vi "Basic.vi"() -> (0 "error out":errorcluster)   [LabVIEW 2019, in "GettingStarted_5785_Host.lvlib"]
uses:
  GettingStarted_5785_Host.lvlib
  <vilib>/userDefined/Silver/nirio_resource_slv.ctl
  <instrlib>/FlexRIO/API/Host/v1/NI FlexRIO/API/Reference Clock Source.ctl
  Upconversion Mode.ctl
  <instrlib>/FlexRIO/API/Host/v1/NI FlexRIO/API/Configure Reference Clock.vi
  <instrlib>/FlexRIO/API/Host/v1/NI FlexRIO/API/Get Property Reference - Fpga Small.vi
  <instrlib>/FlexRIO/API/Host/v1/NI FlexRIO/API/Configure Analog Start Trigger.vi
  <instrlib>/FlexRIO/API/Host/v1/NI FlexRIO/API/Configure Digital Edge Start Trigger.vi
  <instrlib>/FlexRIO/API/Host/v1/NI FlexRIO/API/Configure Immediate Start Trigger.vi
  <instrlib>/FlexRIO/API/Host/v1/NI FlexRIO/API/Read Stream 1D WDT.vi
  <vilib>/measure/matone.llb/Extract Single Tone Information N Chan (CDB).vi
  <vilib>/measure/maspectr.llb/FFT Power Spectrum and PSD for N Chan (CDB).vi
  <vilib>/FPGAPlugInAG/Dynamic/niLvFpga_Close_Dynamic.vi
  <vilib>/rvi/interface/nirviCloseFPGA/nirviCloseFPGA.xnode
  <instrlib>/FlexRIO/API/Host/v1/NI FlexRIO API v1.lvlib
  <resource>/objmgr/niflexrioapiStream.rc
  <vilib>/measure/NI_MAPro.lvlib
panel:
  in  "DUC Freq Shift (Hz)":dbl format="%#_4p"
  in  "DDC Freq Shift (Hz)":dbl format="%#_4p"
  in  "IQ Enabled":bool
  in  "DDC Enabled":bool
  in  "processing mode":T1=enum."None, Two Channels"
  out "AO num Samples":i32=160
  in  "waveform config":T2(array[cluster])=[{"Frequency (Hz)"=500000000.0, "Amplitude (V)"=0.2, "Phase (Deg)"=0.0}, {"Frequency (Hz)"=500000000.0, "Amplitude (V)"=0.20000000000000004, "Phase (Deg)"=0.0}] {"Phase (Deg)" format="%.2p"; "Amplitude (V)" format="%0.2p"; "Frequency (Hz)" format="%0.2p"}
  in  "reference clock source":T3 items=["Default", "Onboard", "PXI_Clk10", "External", "None", "Baseboard Reference"]
  in  "Update Waveform":bool caption="Download AO Waveforms"
  out "Sample Rate":dbl=3200000000.0 format="%#_6p"
  in  "ADC Interleaving Factor":i32=1 min=0 max=2 step=1
  in  "AI num samples":u64=320 step=32
  in  "AI channels":string="AI0,AI1"
  out "Device Power":dbl(slide)=32.59 scale=-1.0..58.0 scale format="%#_3p"
  out "FPGA Temperature":dbl(slide)=48.0 scale=0.0..100.0 scale format="%#_3p"
  in  "Trigger Type":enum32{"Immediate", "Analog", "Digital"}(tab)
  in  "trigger channel":string="AI0"
  in  "rising edge?":bool=TRUE
  in  "level (V)":dbl format="%#_3p"
  in  "hysteresis (V)":dbl=0.01 format="%#_3p"
  in  "digital trigger source":string(combo)
  in  "stop":bool
  in  "Bitfile path":path=path "C:/Repos/bsherman-sandbox/CogRF/5785 Measurements/Common/Original 5785 Example/FPGA Bitfiles/PXIe_5785_KU060.lvbitx"
  in  "Waveform Tab Control":T4(tab)
  out "Waveform Graph":waveform(dbl)[](graph)=[{"t0"=timestamp(0 s since 1904-01-01), "dt"=3.125e-10, "Y"=array[320 elements]}, {"t0"=timestamp(0 s since 1904-01-01), "dt"=3.125e-10, "Y"=array[320 elements]}]
  out "FFT":cluster{"f0":dbl, "df":dbl, "magnitude":dbl[]}[](graph) caption="Waveform Graph"
  out "detected frequencies":dbl[](array[numeric])=[555552707.7834543, 1412702117.9341562] format="%_4p"
  out "AO Out":waveform(dbl)[](graph)=[{"t0"=timestamp(0 s since 1904-01-01), "dt"=3.125e-10, "Y"=[0.0, 0.16629392246050906, 0.1847759065022574, 0.03901806440322561, -0.1414213562373095, -0.19615705608064604, -0.07653668647301802, 0.11111404660392049, 0.2, 0.11111404660392035, -0.07653668647301787, -0.19615705608064607, -0.14142135623730956, 0.03901806440322578, 0.18477590650225734, 0.16629392246050892, 0.0, -0.16629392246050909, -0.18477590650225734, -0.03901806440322547, 0.14142135623730956, 0.196157056080646, 0.07653668647301785, -0.11111404660392055, -0.19999999999999996, -0.11111404660392023, 0.07653668647301798, 0.19615705608064604, 0.1414213562373094, -0.03901806440322589, -0.18477590650225728, -0.1662939224605088, 5.551115123125783e-17, 0.16629392246050909, 0.18477590650225723, 0.03901806440322533, -0.14142135623730945, -0.19615705608064585, -0.07653668647301788, 0.11111404660392057, 0.1999999999999999, 0.11111404660392012, -0.07653668647301798, -0.196157056080646, -0.14142135623730936, 0.03901806440322589, 0.18477590650225725, 0.16629392246050878, -2.7755575615628914e-17, -0.16629392246050906, -0.18477590650225725, -0.03901806440322536, 0.14142135623730942, 0.19615705608064593, 0.07653668647301794, -0.11111404660392066, -0.1999999999999999, -0.11111404660392014, 0.07653668647301792, 0.19615705608064604, 0.14142135623730945, -0.039018064403225916, -0.18477590650225728, -0.1662939224605088, 0.0, 0.16629392246050914, 0.18477590650225728, 0.03901806440322533, -0.14142135623730945, -0.19615705608064596, -0.07653668647301792, 0.11111404660392063, 0.1999999999999999, 0.11111404660392017, -0.07653668647301792, -0.1961570560806461, -0.14142135623730945, 0.039018064403226, 0.18477590650225728, 0.1662939224605088, 0.0, -0.1662939224605092, -0.18477590650225728, -0.039018064403225305, 0.14142135623730945, 0.196157056080646, 0.07653668647301792, -0.11111404660392071, -0.1999999999999999, -0.11111404660392012, 0.07653668647301792, 0.19615705608064615, 0.14142135623730945, -0.039018064403226055, -0.18477590650225728, -0.1662939224605088, 0.0, 0.16629392246050925, 0.18477590650225728, 0.039018064403225305, -0.14142135623730945, -0.19615705608064601, -0.07653668647301792, 0.11111404660392074, 0.1999999999999999, 0.11111404660392014, -0.07653668647301792, -0.1961570560806461, -0.14142135623730945, 0.03901806440322597, 0.18477590650225728, 0.1662939224605088, 0.0, -0.16629392246050914, -0.18477590650225728, -0.03901806440322539, 0.14142135623730945, 0.196157056080646, 0.07653668647301792, -0.1111140466039206, -0.1999999999999999, -0.11111404660392023, 0.07653668647301792, 0.19615705608064604, 0.14142135623730945, -0.03901806440322583, -0.18477590650225728, -0.16629392246050886, 0.0, 0.16629392246050909, 0.18477590650225728, 0.03901806440322539, -0.14142135623730945, -0.19615705608064593, -0.07653668647301792, 0.1111140466039206, 0.1999999999999999, 0.11111404660392019, -0.07653668647301792, -0.19615705608064607, -0.14142135623730945, 0.039018064403225944, 0.18477590650225728, 0.1662939224605088, 0.0, -0.16629392246050914, -0.18477590650225728, -0.03901806440322533, 0.14142135623730945, 0.19615705608064596, 0.07653668647301792, -0.11111404660392063, -0.1999999999999999, -0.11111404660392017, 0.07653668647301792, 0.1961570560806461, 0.14142135623730945, -0.039018064403226, -0.18477590650225728, -0.1662939224605088]}, {"t0"=timestamp(0 s since 1904-01-01), "dt"=3.125e-10, "Y"=[0.0, 0.16629392246050909, 0.1847759065022574, 0.03901806440322561, -0.1414213562373095, -0.19615705608064612, -0.07653668647301798, 0.11111404660392046, 0.20000000000000004, 0.11111404660392046, -0.076536686473018, -0.19615705608064612, -0.1414213562373095, 0.03901806440322561, 0.1847759065022574, 0.1662939224605091, 0.0, -0.166293922460509, -0.1847759065022574, -0.03901806440322575, 0.1414213562373095, 0.1961570560806461, 0.07653668647301802, -0.11111404660392044, -0.2, -0.11111404660392044, 0.07653668647301787, 0.1961570560806461, 0.14142135623730956, -0.03901806440322575, -0.18477590650225734, -0.16629392246050897, 0.0, 0.16629392246050903, 0.18477590650225734, 0.03901806440322558, -0.14142135623730956, -0.196157056080646, -0.07653668647301785, 0.11111404660392044, 0.19999999999999996, 0.11111404660392034, -0.07653668647301798, -0.196157056080646, -0.1414213562373094, 0.039018064403225666, 0.18477590650225728, 0.16629392246050895, -5.551115123125783e-17, -0.166293922460509, -0.18477590650225723, -0.039018064403225555, 0.14142135623730945, 0.19615705608064596, 0.07653668647301788, -0.11111404660392041, -0.1999999999999999, -0.11111404660392037, 0.07653668647301798, 0.196157056080646, 0.14142135623730936, -0.03901806440322561, -0.18477590650225725, -0.16629392246050897, 2.7755575615628914e-17, 0.16629392246050897, 0.18477590650225725, 0.03901806440322564, -0.14142135623730942, -0.19615705608064601, -0.07653668647301794, 0.11111404660392041, 0.1999999999999999, 0.11111404660392041, -0.07653668647301792, -0.19615705608064601, -0.14142135623730945, 0.03901806440322564, 0.18477590650225728, 0.16629392246050897, 0.0, -0.16629392246050897, -0.18477590650225728, -0.03901806440322564, 0.14142135623730945, 0.19615705608064601, 0.07653668647301792, -0.11111404660392041, -0.1999999999999999, -0.11111404660392041, 0.07653668647301792, 0.19615705608064601, 0.14142135623730945, -0.03901806440322564, -0.18477590650225728, -0.16629392246050897, 0.0, 0.16629392246050897, 0.18477590650225728, 0.03901806440322564, -0.14142135623730945, -0.19615705608064601, -0.07653668647301792, 0.11111404660392041, 0.1999999999999999, 0.11111404660392041, -0.07653668647301792, -0.19615705608064601, -0.14142135623730945, 0.03901806440322564, 0.18477590650225728, 0.16629392246050897, 0.0, -0.16629392246050897, -0.18477590650225728, -0.03901806440322564, 0.14142135623730945, 0.19615705608064601, 0.07653668647301792, -0.11111404660392041, -0.1999999999999999, -0.11111404660392041, 0.07653668647301792, 0.19615705608064601, 0.14142135623730945, -0.03901806440322564, -0.18477590650225728, -0.16629392246050897, 0.0, 0.16629392246050897, 0.18477590650225728, 0.03901806440322564, -0.14142135623730945, -0.19615705608064601, -0.07653668647301792, 0.11111404660392041, 0.1999999999999999, 0.11111404660392041, -0.07653668647301792, -0.19615705608064601, -0.14142135623730945, 0.03901806440322564, 0.18477590650225728, 0.16629392246050897, 0.0, -0.16629392246050897, -0.18477590650225728, -0.03901806440322564, 0.14142135623730945, 0.19615705608064601, 0.07653668647301792, -0.11111404660392041, -0.1999999999999999, -0.11111404660392041, 0.07653668647301792, 0.19615705608064601, 0.14142135623730945, -0.03901806440322564, -0.18477590650225728, -0.16629392246050897]}] caption="Waveform Graph"
  out "Limit (W)":dbl=58.0
  out "Power (W)":dbl=32.59
  out "Limit (C)":dbl=96.0
  out "Temp (C)":dbl=48.0 format="%#_4p"
  in  "RIO Device":T5="5785_00"
  # "Overview: Configure an acquisition for a FlexRIO target and transfer the data to the host using the FlexRIO Host API.  Loop an output waveform\nRequirements: FlexRIO\nInstructions: \n 1. Loop AI channels back to AO channels using SMA cables\n 2. Select the RIO Device that corresponds to the FlexRIO target. \n 3. Select the bitfile path that corresponds to your device\n 4. Optionally configure the clocking, stream, and trigger. \n 5. Run the VI"
  # "Resource Configuration"
  # "Clocking configuration"
  # "Input Waveform Configuration"
  # "Device Monitoring"
  # "Output Waveform Configuration"
  # "Digital Upconverter Configuration"
  # "Frequency (Hz)"
  # "Amplitude (V)"
  # "Phase (Deg)"
  # "AO 0"
  # "AO 1"
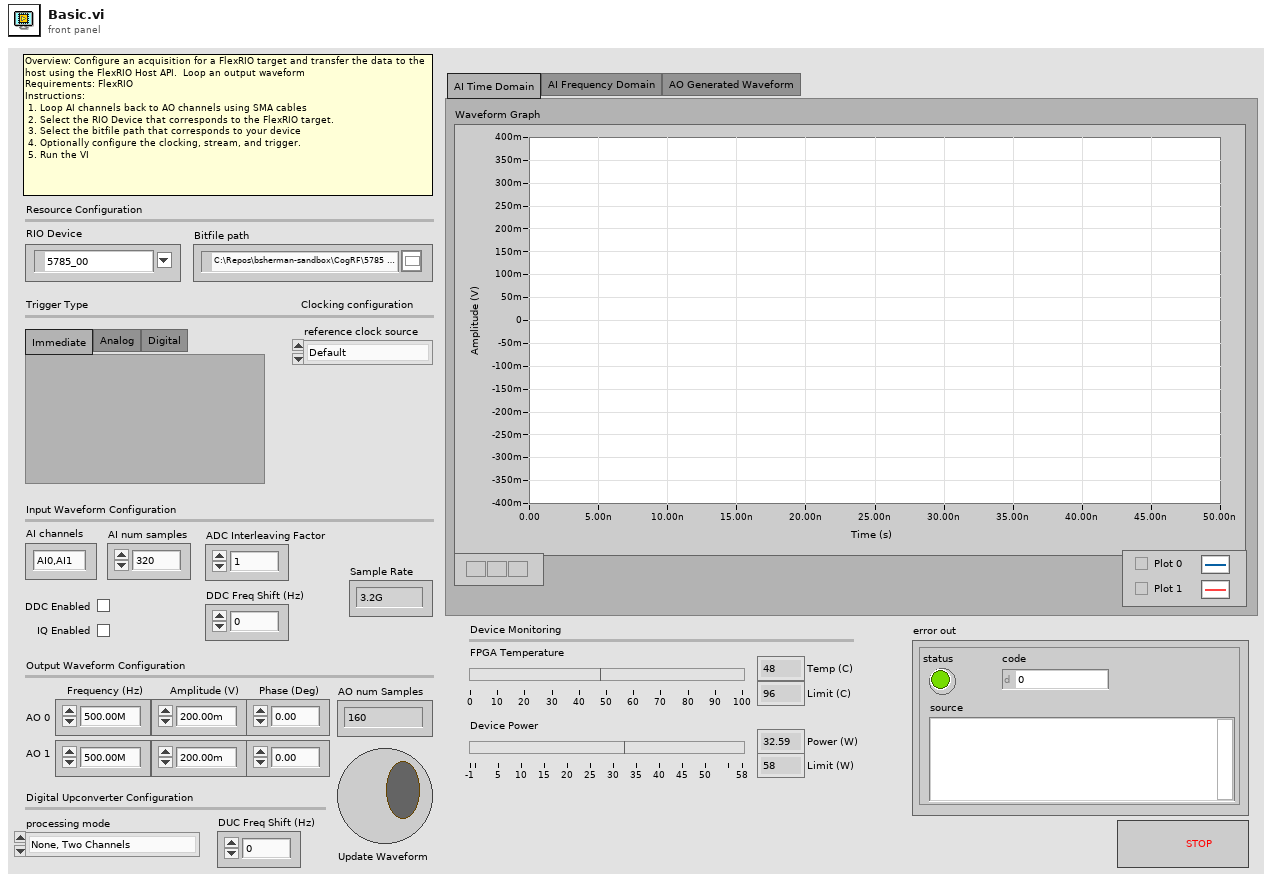
[diagram p1: front panel]
types:
  T1 = typedef "GettingStarted_5785_Host.lvlib/Upconversion Mode.ctl" = enum16{"None, One Channel", "None, Two Channels", "FPGA-only, One Channel", "DAC and FPGA, One Channel", "DAC-only, One Channel"}
  T2 = cluster{"Frequency (Hz)":dbl, "Amplitude (V)":dbl, "Phase (Deg)":dbl}[]
  T3 = typedef "NI FlexRIO API v1.lvlib/Reference Clock Source.ctl" = i32
  T4 = enum32{"AI Time Domain", "AI Frequency Domain", "AO Generated Waveform"}
  T5 = typedef "nirio_resource_slv.ctl" = tag
  T6 = cluster{"averaging mode":enum16{"No averaging", "Vector averaging", "RMS averaging", "Peak hold"}, "weighting mode":enum16{"Linear", "Exponential"}, "number of averages":u32}
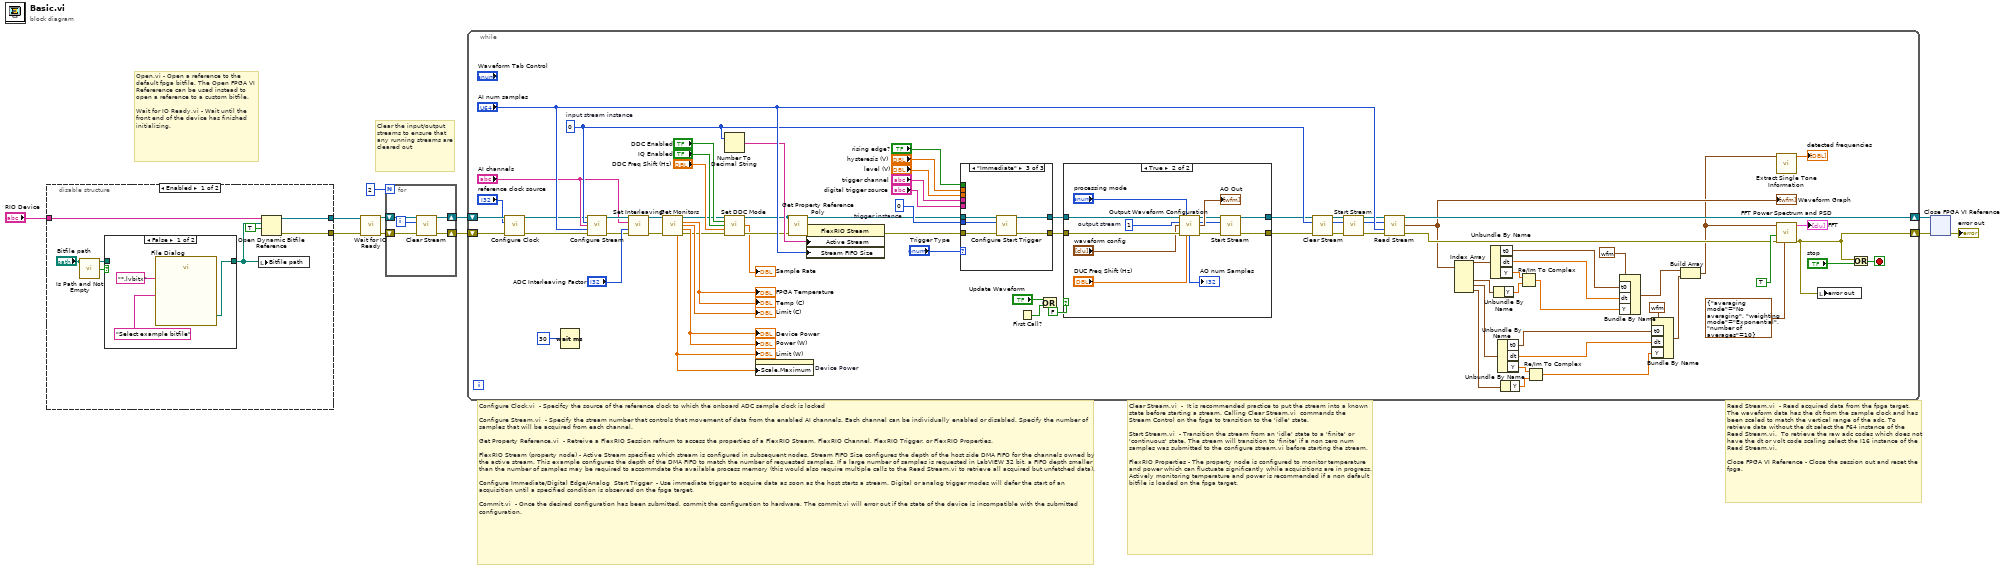
[diagram p0: block diagram]
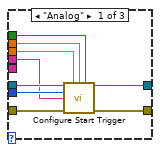
[diagram p3: hidden frame]
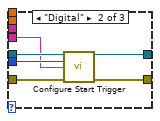
[diagram p4: hidden frame]
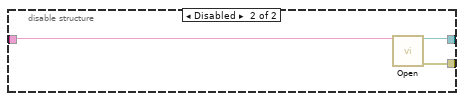
[diagram p6: hidden frame]
diagram:
  # "Clear the input/output\nstreams to ensure that\nany running streams are cleared out"
  # "Read Stream.vi  - Read acquired data from the fpga target. The waveform data has the dt from the sample clock and has been scaled to match the vertical range of the adc. To retrieve data without the dt select the F64 instance of the Read Stream.vi.  To retrieve the raw adc codes which does not have the dt or volt code scaling select the I16 instance of the Read Stream.vi.  \n\nClose FPGA VI Reference - Close the session out and reset the fpga."
  # "Clear Stream.vi  -  It is recommended practice to put the stream into a known state before starting a stream. Calling Clear Stream.vi  commands the Stream Control on the fpga to transition to the 'idle' state.\n\nStart Stream.vi  - Transition the stream from an 'idle' state to a 'finite' or 'continuous' state. The stream will transition to 'finite' if a non zero num samples was submitted to the configure stream.vi before starting the stream.  \n\nFlexRIO Properties - The property node is configured to monitor temperature and power which can fluctuate significantly while acquisitions are in progress. Actively monitoring temperature and power is recommended if a non default bitfile is loaded on the fpga target."
  # "Configure Clock.vi  - Specifcy the source of the reference clock to which the onboard ADC sample clock is locked\n\nConfigure Stream.vi  - Specify the stream number that controls that movement of data from the enabled AI channels. Each channel can be individually enabled or disabled. Specify the number of samples that will be acquired from each channel. \n\nGet Property Reference.vi  - Retreive a FlexRIO Session refnum to access the properties of a FlexRIO Stream, FlexRIO Channel, FlexRIO Trigger, or FlexRIO Properties.\n\nFlexRIO Stream (property node) - Active Stream specifies which stream is configured in subsequent nodes. Stream FIFO Size configures the depth of the host side DMA FIFO for the channels owned by the active stream. This example configures the depth of the DMA FIFO to match the number of requested samples. If a large number of samples is requested in LabVIEW 32 bit, a FIFO depth smaller than the number of samples may be required to accommdate the available process memory (this would also require multiple calls to the Read Stream.vi to retrieve all acquired but unfetched data). \n\nConfigure Immediate/Digital Edge/Analog  Start Trigger  - Use immediate trigger to acquire data as soon as the host starts a stream. Digital or analog trigger modes will defer the start of an acquisition until a specified condition is observed on the fpga target. \n\nCommit.vi  - Once the desired configuration has been submitted, commit the configuration to hardware. The commit.vi will error out if the state of the device is incompatible with the submitted configuration."
  # "Open.vi - Open a reference to the default fpga bitfile. The Open FPGA VI Refererence can be used instead to open a reference to a custom bitfile.\n\nWait for IO Ready.vi - Wait until the front end of the device has finished initializing."
  n1 = disable-structure shown="Enabled" {
    disable-tunnel: [w18 w25] -> w10
    disable-tunnel: [w17 w24] -> w9
    disable-tunnel: "RIO Device" -> [w16 w23]
    frame Enabled {
      n2 = call <vilib>:"Is Path and Not Empty.vi"("path"="Bitfile path") -> ("Is Path and Not Empty?"=w13:bool)  [unwired: 4 in]
      n3 = case shown="False" w13 {
        tunnel: "Bitfile path" -> [_ w22]
        tunnel: [w20 w22] -> w12
        frame False {
          n4 = call "File Dialog"("prompt"="Select example bitfile", "pattern (all files)"="*.lvbitx") -> ("selected path"=w20:path)  [unwired: 10 in, 3 out]
        }
        frame True {
        }
      }
      n5 = local write "Bitfile path"(w12) -> ()
      n6 = Open Dynamic Bitfile Reference(0:w16, 1:w12, 2:TRUE ("Run When Loaded")) -> (5:w17:refnum<k20>, 8:w18:errorcluster)  [unwired: 2 in]
    }
    frame Disabled {
      n7 = call <instrlib>:"Open.vi"("RIO Device"=w23) -> ("fpga interface out"=w24:refnum<k20>, "error out"=w25:errorcluster)  [unwired: 13 in]
    }
  }
  n8 = call <instrlib>:"Wait for IO Ready.vi"("fpga interface in"=w9, "error in"=w10) -> ("fpga interface out"=w5:refnum<k20>, "error out"=w4:errorcluster)  [unwired: 10 in, 2 out]
  n9 = for {
    N: 2 -> [_]
    shift-right: [w27] -> w2
    shift-left: w5 -> [w30]
    shift-right: [w28] -> w3
    shift-left: w4 -> [w29]
    i -> [w26]
    n10 = call <instrlib>:"Clear Stream.vi"("fpga interface in"=w30, "stream instance"=w26, "error in"=w29) -> ("fpga interface out"=w27:refnum<k20>, "error out"=w28:errorcluster)  [unwired: 10 in, 1 out]
  }
  n11 = while {
    shift-right: [w66] -> w6
    shift-left: w3 -> [w109]
    shift-right: [w107] -> w7
    shift-left: w2 -> [w108]
    stop <- w75 stop-if-true
    w98 = u32 0  # trigger instance
    w94 = u32 0  # input stream instance
    n12 = call-poly <instrlib>:"Configure Clock.vi"("fpga interface in"=w108, "reference clock source"="reference clock source", "error in"=w109) -> ("fpga interface out"=w69:refnum<k20>, "error out"=w102:errorcluster)  [unwired: 11 in]
    n13 = Wait (ms)(milliseconds to wait=u32 30) -> ()  [unwired: 1 out]
    n14 = call <instrlib>:"Configure Stream.vi"("fpga interface in"=w69, "stream instance"=w94, "channels enabled"="AI channels", "num samples"="AI num samples", "error in"=w102) -> ("fpga interface out"=w92:refnum<k20>, "error out"=w90:errorcluster)  [unwired: 7 in, 2 out]
    n15 = call "Set Interleaving.vi"("fpga interface in"=w92, "AI channels enabled"="AI channels", "ADC Interleaving Factor"="ADC Interleaving Factor", "error in (no error)"=w90) -> ("fpga interface out"=w71:refnum<k20>, "error out"=w70:errorcluster)  [unwired: 10 in]
    n16 = call "Get Monitors.vi"("fpga interface in"=w71, "error in (no error)"=w70) -> ("fpga interface out"=w58:refnum<k20>, "FPGA Temperature (C)"=→"Temp (C)" →"FPGA Temperature":dbl, "Temperature Limit (C)"=→"Limit (C)":dbl, "Total Power (W)"=→"Power (W)" →"Device Power":dbl, "Power Limit (W)"=w84:dbl, "error out"=w57:errorcluster)  [unwired: 8 in]
    "Limit (W)" <- w84
    n17 = Number To Decimal String(number=w94) -> (decimal integer string=w100:string)  [unwired: 1 in]
    n18 = call "Set DDC Mode.vi"("fpga refnum"=w58, "DDC Enabled"="DDC Enabled", "IQ Enabled"="IQ Enabled", "DDC Frequency Shift (Hz)"="DDC Freq Shift (Hz)", "error in (no error)"=w57) -> ("fpga refnum out"=w59:refnum<k20>, "sample rate"=→"Sample Rate":dbl, "error out"=w60:errorcluster)  [unwired: 8 in]
    n19 = property on="Device Power" class="Slide (strict)"("Scale.Maximum"=w84) -> ()  [unwired: 2 in, 2 out]
    n20 = call-poly <instrlib>:"Get Property Reference Poly.vi"("error in (no error)"=w60, "fpga interface in"=w59) -> ("error out"=w89:errorcluster, "property reference"=w88:refnum<k20>)  [unwired: 4 in, 1 out]
    n21 = property class="FlexRIO Stream"(reference=w88, error in=w89, "Active Stream"=w100, "Stream FIFO Size"="AI num samples") -> (error out=w97:errorcluster)  [unwired: 1 out]
    n22 = case shown="\"Immediate\"" "Trigger Type" {
      tunnel: w59 -> [w133 w139 w144]
      tunnel: w97 -> [w132 w138 w143]
      tunnel: [w131 w137 w142] -> w96
      tunnel: [w130 w136 w141] -> w95
      tunnel: w98 -> [w129 w135 w140]
      tunnel: "trigger channel" -> [w128 _ _]
      tunnel: "level (V)" -> [w127 _ _]
      tunnel: "hysteresis (V)" -> [w126 _ _]
      tunnel: "rising edge?" -> [w125 _ _]
      tunnel: "digital trigger source" -> [_ w134 _]
      frame "Analog" {
        n23 = call-poly <instrlib>:"Configure Start Trigger.vi"("fpga interface in"=w133, "level"=w127, "hysteresis"=w126, "rising edge?"=w125, "trigger instance"=w129, "channel"=w128, "error in"=w132) -> ("fpga interface out"=w131:refnum<k20>, "error out"=w130:errorcluster)  [unwired: 6 in, 1 out]
      }
      frame "Digital" {
        n24 = call-poly <instrlib>:"Configure Start Trigger.vi"("fpga interface in"=w139, "trigger instance"=w135, "trigger source"=w134, "error in"=w138) -> ("fpga interface out"=w137:refnum<k20>, "error out"=w136:errorcluster)  [unwired: 9 in, 1 out]
      }
      frame "Immediate" {
        n25 = call-poly <instrlib>:"Configure Start Trigger.vi"("fpga interface in"=w144, "trigger instance"=w140, "error in"=w143) -> ("fpga interface out"=w142:refnum<k20>, "error out"=w141:errorcluster)  [unwired: 10 in, 1 out]
      }
    }
    n26 = First Call?() -> (First Call?: T/F=w53:bool)
    n27 = Or(x="Update Waveform", y=w53) -> ()  [unwired: 1 out]
    n28 = case shown="True" FALSE {
      tunnel: [w111 w124] -> w65
      tunnel: [w110 w123] -> w64
      tunnel: w96 -> [w111 w121]
      tunnel: w95 -> [w110 w120]
      frame False {
      }
      frame True {
        w117 = u32 1  # output stream
        n29 = call "Output Waveform Configuration.vi"("Refnum in"=w121, "processing mode"="processing mode", "output stream instance"=w117, "waveform config"="waveform config", "error in (no error)"=w120, "DUC Frequency Shift"="DUC Freq Shift (Hz)") -> ("Refnum out"=w118:refnum<k20>, "output stream instance out"=w116:u32, "waveforms out"=→"AO Out":waveform(dbl)[], "ao wfm samples"=→"AO num Samples":i32, "error out"=w119:errorcluster)  [unwired: 5 in]
        n30 = call <instrlib>:"Start Stream.vi"("fpga interface in"=w118, "stream instance"=w116, "error in"=w119) -> ("fpga interface out"=w124:refnum<k20>, "error out"=w123:errorcluster)  [unwired: 10 in, 1 out]
      }
    }
    n31 = call <instrlib>:"Clear Stream.vi"("fpga interface in"=w65, "stream instance"=w94, "error in"=w64) -> ("fpga interface out"=w82:refnum<k20>, "stream instance out"=w81:u32, "error out"=w80:errorcluster)  [unwired: 10 in]
    n32 = call <instrlib>:"Start Stream.vi"("fpga interface in"=w82, "stream instance"=w81, "error in"=w80) -> ("fpga interface out"=w73:refnum<k20>, "stream instance out"=w79:u32, "error out"=w72:errorcluster)  [unwired: 10 in]
    n33 = call-poly <instrlib>:"Read Stream.vi"("fpga interface in"=w73, "stream instance"=w79, "samples"="AI num samples", "error in"=w72) -> ("fpga interface out"=w107:refnum<k20>, "read data"=w50:waveform(dbl)[], "error out"=w76:errorcluster)  [unwired: 7 in, 2 out]
    "Waveform Graph" <- w50
    n34 = Index Array(array=w50) -> (element #1=w49:waveform(dbl), element #2=w48:waveform(dbl), element #3=w38:waveform(dbl), element #4=w37:waveform(dbl))  [unwired: 4 in]
    n35 = Unbundle By Name(w49) -> ("t0"=w46:timestamp, "dt"=w45:dbl, "Y"=w44:dbl[])
    n36 = Unbundle By Name(w48) -> ("Y"=w43:dbl[])
    n37 = Unbundle By Name(w38) -> ("t0"=w34:timestamp, "dt"=w35:dbl, "Y"=w39:dbl[])
    n38 = Unbundle By Name(w37) -> ("Y"=w40:dbl[])
    n39 = Re/Im To Complex(1:w43, 2:w44) -> (0:w42:cdb[])
    n40 = Re/Im To Complex(1:w40, 2:w39) -> (0:w36:cdb[])
    n41 = Bundle By Name(cluster=waveform(cdb) {"t0"=timestamp(0 s since 1904-01-01), "dt"=1.0, "Y"=[]} ("Waveform"), "t0"=w46, "dt"=w45, "Y"=w42) -> (w33:waveform(cdb))
    n42 = Bundle By Name(cluster=waveform(cdb) {"t0"=timestamp(0 s since 1904-01-01), "dt"=1.0, "Y"=[]} ("Waveform"), "t0"=w34, "dt"=w35, "Y"=w36) -> (w32:waveform(cdb))
    n43 = Build Array(w33, w32) -> (w31:waveform(cdb)[])
    n44 = call-poly <vilib>:"Extract Single Tone Information.vi"("time signals in"=w31) -> ("detected frequencies"=→"detected frequencies":dbl[])  [unwired: 5 in, 5 out]
    n45 = call-poly <vilib>:"FFT Power Spectrum and PSD.vi"("averaging parameters"=T6 {"averaging mode"=enum."No averaging", "weighting mode"=enum."Exponential", "number of averages"=10}, "error in (no error)"=w76, "dB On (F)"=TRUE, "time signals"=w31) -> ("error out"=w66:errorcluster, "Power Spectrum / PSD"=→"FFT":cluster{"f0":dbl, "df":dbl, "magnitude":dbl[]}[])  [unwired: 4 in, 2 out]
    n46 = local write "error out"(w66) -> ()
    n47 = Or(x=w66, y="stop") -> (x .or. y?=w75:bool)
  }
  n48 = xnode "Close FPGA VI Reference"("FPGA VI Reference In"=w7, "error in"=w6) -> ("error out"=→"error out":errorcluster)
